vi "5.1 Sub-VI.vi"(11 "data":u16) -> (3 "String":string)   [LabVIEW 2014]
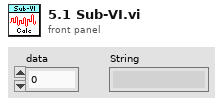
[diagram p1: front panel]
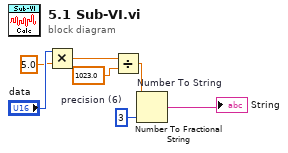
[diagram p0: block diagram]
diagram:
  w4 = i16 3  # precision (6)
  n1 = Multiply(x="data", y=5.0) -> (x*y=w2:dbl)
  n2 = Divide(x=w2, y=1023.0 ("x")) -> (x/y=w5:dbl)
  n3 = Number To Fractional String "Number To String"(number=w5, precision (6)=w4) -> (F-format string=→"String":string)  [unwired: 2 in]
